vi "Get Control Attribute Value From Ini File.vi"(6 "AttributeType":variant, 7 "Section Name":string, 8 "error in (no error)":errorcluster, 9 "AttributeValue":variant, 10 "AttributeNames":string, 11 "Ini Config Ref":T1) -> (0 "error out":errorcluster, 1 "AttributeValue Out":variant, 2 "AttributeNames Out":string, 3 "Ini Config Ref Out":T1)   [LabVIEW 2015, in "UIConfiguration.lvclass"]
uses:
  UIConfiguration.lvclass
  <vilib>/Utility/config.llb/Config Data RefNum.ctl
  <vilib>/Utility/config.llb/Read Key (String).vi
  <vilib>/Utility/config.llb/Read Key (U32).vi
  <vilib>/Utility/config.llb/NI_LVConfig.lvlib
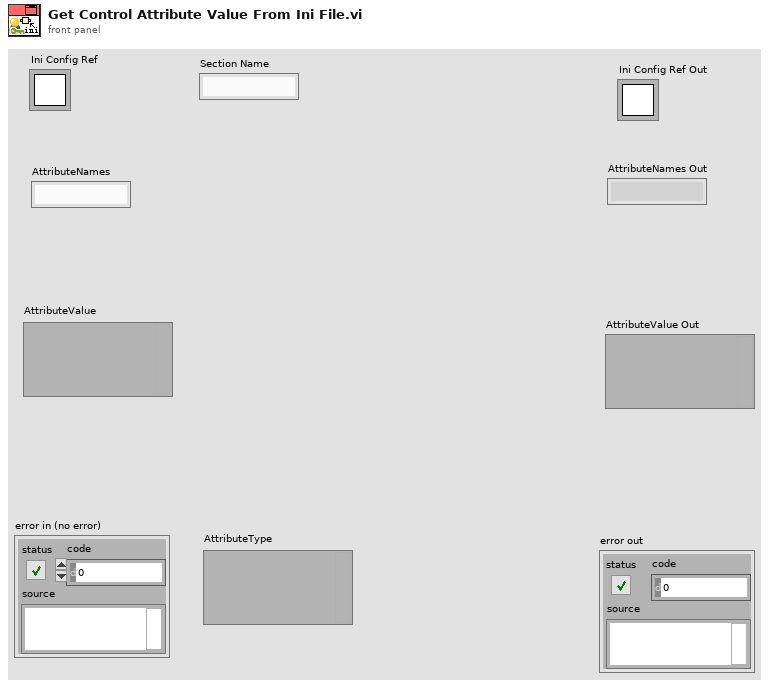
[diagram p1: front panel]
types:
  T1 = typedef "NI_LVConfig.lvlib/Config Data RefNum.ctl" = refnum<k1>
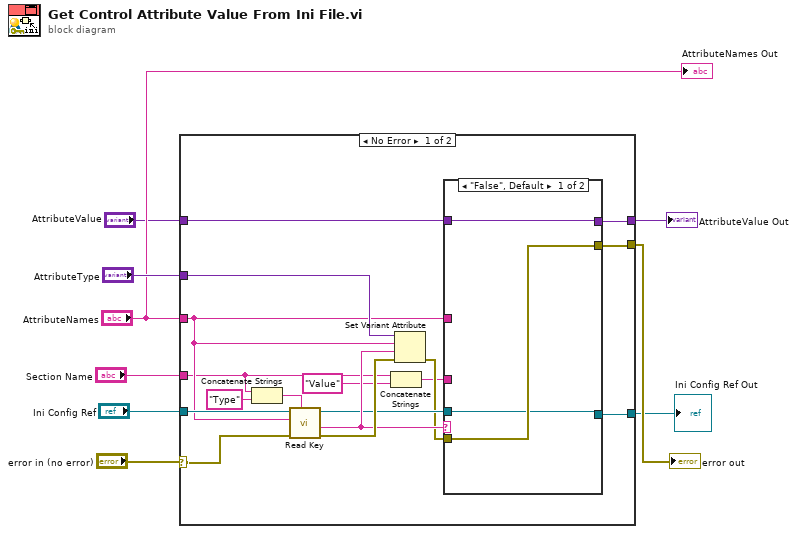
[diagram p0: block diagram]
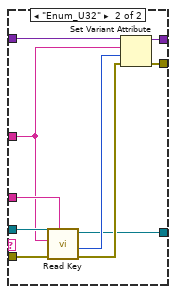
[diagram p2: hidden frame]
diagram:
  n1 = case shown="No Error" "error in (no error)" {
    selector: "error in (no error)" -> [w25 w41]
    tunnel: "AttributeType" -> [w22 _]
    tunnel: "Ini Config Ref" -> [w26 w40]
    tunnel: "Section Name" -> [w15 _]
    tunnel: "AttributeNames" -> [w16 _]
    tunnel: [w12 w42] -> w5
    tunnel: [w11 w41] -> w4
    tunnel: "AttributeValue" -> [w19 w42]
    tunnel: [w10 w40] -> w1
    frame No Error {
      n2 = Concatenate Strings(w15, "Type" ("string")) -> (w23:string)
      n3 = call-poly <vilib>:"Read Key.vi"("section"=w23, "error in (no error)"=w25, "key"=w16, "refnum"=w26) -> ("error out"=w21:errorcluster, "value"=w20:string, "refnum out"=w18:T1)  [unwired: 4 in, 1 out]
      n4 = Concatenate Strings(w15, "Value" ("string")) -> (w13:string)
      n5 = Set Variant Attribute(Variant=w22, name=w16, value=w20, error in=w21) -> (error out=w17:errorcluster)  [unwired: 2 out]
      n6 = case shown="\"False\", Default" w20 {
        tunnel: w19 -> [w29 w36]
        tunnel: w18 -> [w27 w39]
        tunnel: w17 -> [w28 w38]
        tunnel: w16 -> [_ w35]
        tunnel: w13 -> [_ w37]
        tunnel: [w29 w32] -> w12
        tunnel: [w28 w31] -> w11
        tunnel: [w27 w30] -> w10
        frame "False", Default {
        }
        frame "Enum_U32" {
          n7 = call-poly <vilib>:"Read Key.vi"("section"=w37, "error in (no error)"=w38, "key"=w35, "refnum"=w39) -> ("error out"=w33:errorcluster, "value"=w34:u32, "refnum out"=w30:T1)  [unwired: 4 in, 1 out]
          n8 = Set Variant Attribute(Variant=w36, name=w35, value=w34, error in=w33) -> (Variant out=w32:variant, error out=w31:errorcluster)  [unwired: 1 out]
        }
      }
    }
    frame Error {
    }
  }
  "AttributeValue Out" <- w5
  "error out" <- w4
  "Ini Config Ref Out" <- w1
  "AttributeNames Out" <- "AttributeNames"
